vi "Volt Reader Trigger12.vi"() -> ()   [LabVIEW 2014]
uses:
  Enum State Machine Typedef.ctl
  <vilib>/Utility/error.llb/DialogType.ctl
  <vilib>/_DAQmxBase/Internals/DAQmxBase Create Channel (AI-Voltage-Basic).vi
  <vilib>/_DAQmxBase/Internals/DAQmxBase Timing (Sample Clock).vi
  <vilib>/measure/mamon.llb/Trigger Detection for 1 Channel.vi
  <vilib>/_DAQmxBase/Internals/DAQmxBase Read (Analog 2D DBL NChan NSamp).vi
  <vilib>/measure/NI_MAPro.lvlib
panel:
  out "Raw Graph":waveform(dbl)(graph)
  in  "Center":bool
  in  "Offset (percent of buffer)":dbl(knob) scale=-50.0..50.0
  out "State":T1
  out "Waveform Graph":waveform(dbl)(graph)
  in  "Buffer (Seconds)":dbl
  out "Threshold":dbl
  in  "units":i32(ring)=10348 items=["Volts"=10348, "From Custom Scale"=10065]
  in  "stop":bool
  in  "physical channels":tag
  in  "maximum value":dbl=5.0 format="%0.2f"
  in  "minimum value":dbl=-5.0 format="%0.2f"
  in  "rate":i32=1000 caption="Sample Rate"
  # "The inputs above MUST BE\nPreset before running"
  # "NOTE: Just change the Y axis value"
  # "Make Sure that Buffer does not equal 0"
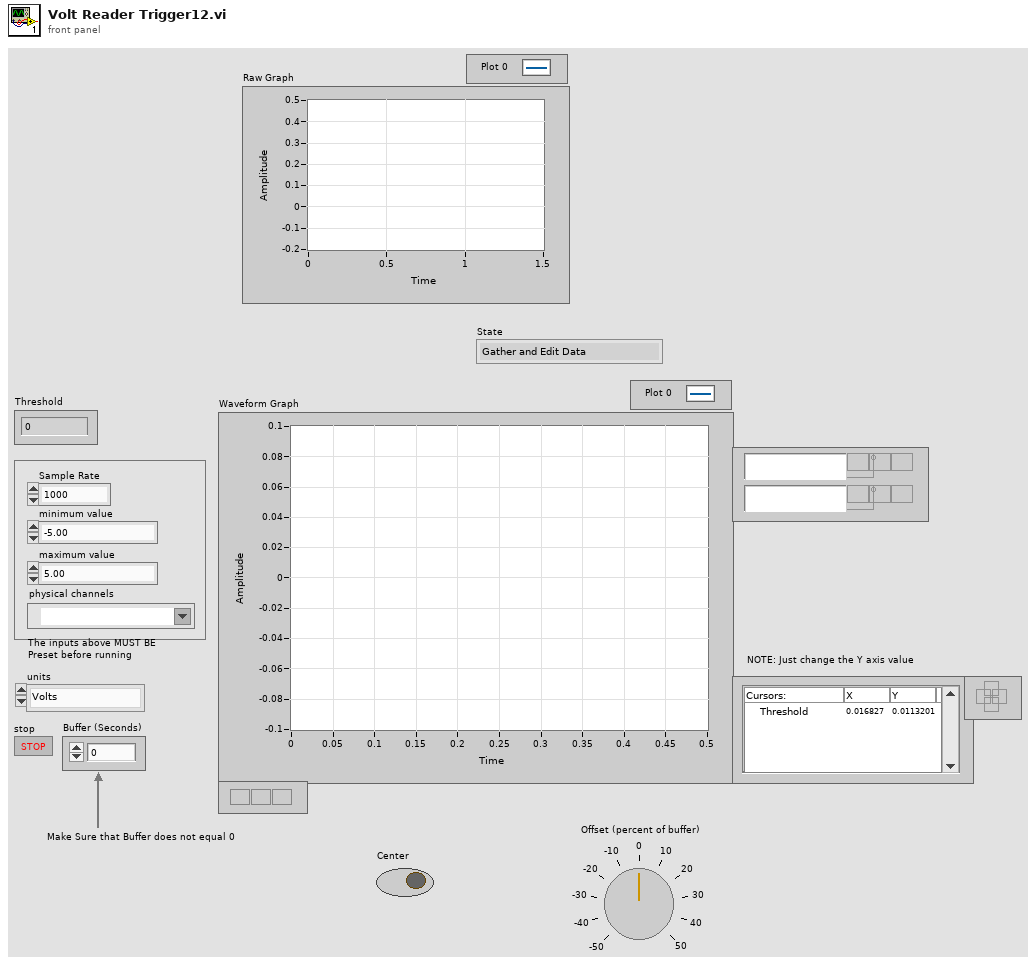
[diagram p1: front panel]
types:
  T1 = typedef "Enum State Machine Typedef.ctl" = enum16{"Gather and Edit Data", "Trigger Occured", "Just Displayed"}
  T2 = typedef "DialogType.ctl" = u16
  T3 = typedef "LVCursorListTypeDef.ctl" = cluster{"Name":string, "Color":u32, "Style":u8, "Point Style":u8, "Name Visible":bool, "Allow Drag":bool, "Cursor Mode":u32, "Plot":i32, "Index":i32, "Position":cluster{"X":dbl, "Y":dbl}, "X Scale":u32, "Y Scale":u32, "Watch Plots":i32[], "Watch All Plots":bool, "Plot Area":i32, "Label Offset":cluster{"X":dbl, "Y":dbl}}[]
  T4 = cluster{"Name":string, "Color":u32, "Style":u8, "Point Style":u8, "Name Visible":bool, "Allow Drag":bool, "Cursor Mode":u32, "Plot":i32, "Index":i32, "Position":cluster{"X":dbl, "Y":dbl}, "X Scale":u32, "Y Scale":u32, "Watch Plots":i32[], "Watch All Plots":bool, "Plot Area":i32, "Label Offset":cluster{"X":dbl, "Y":dbl}}
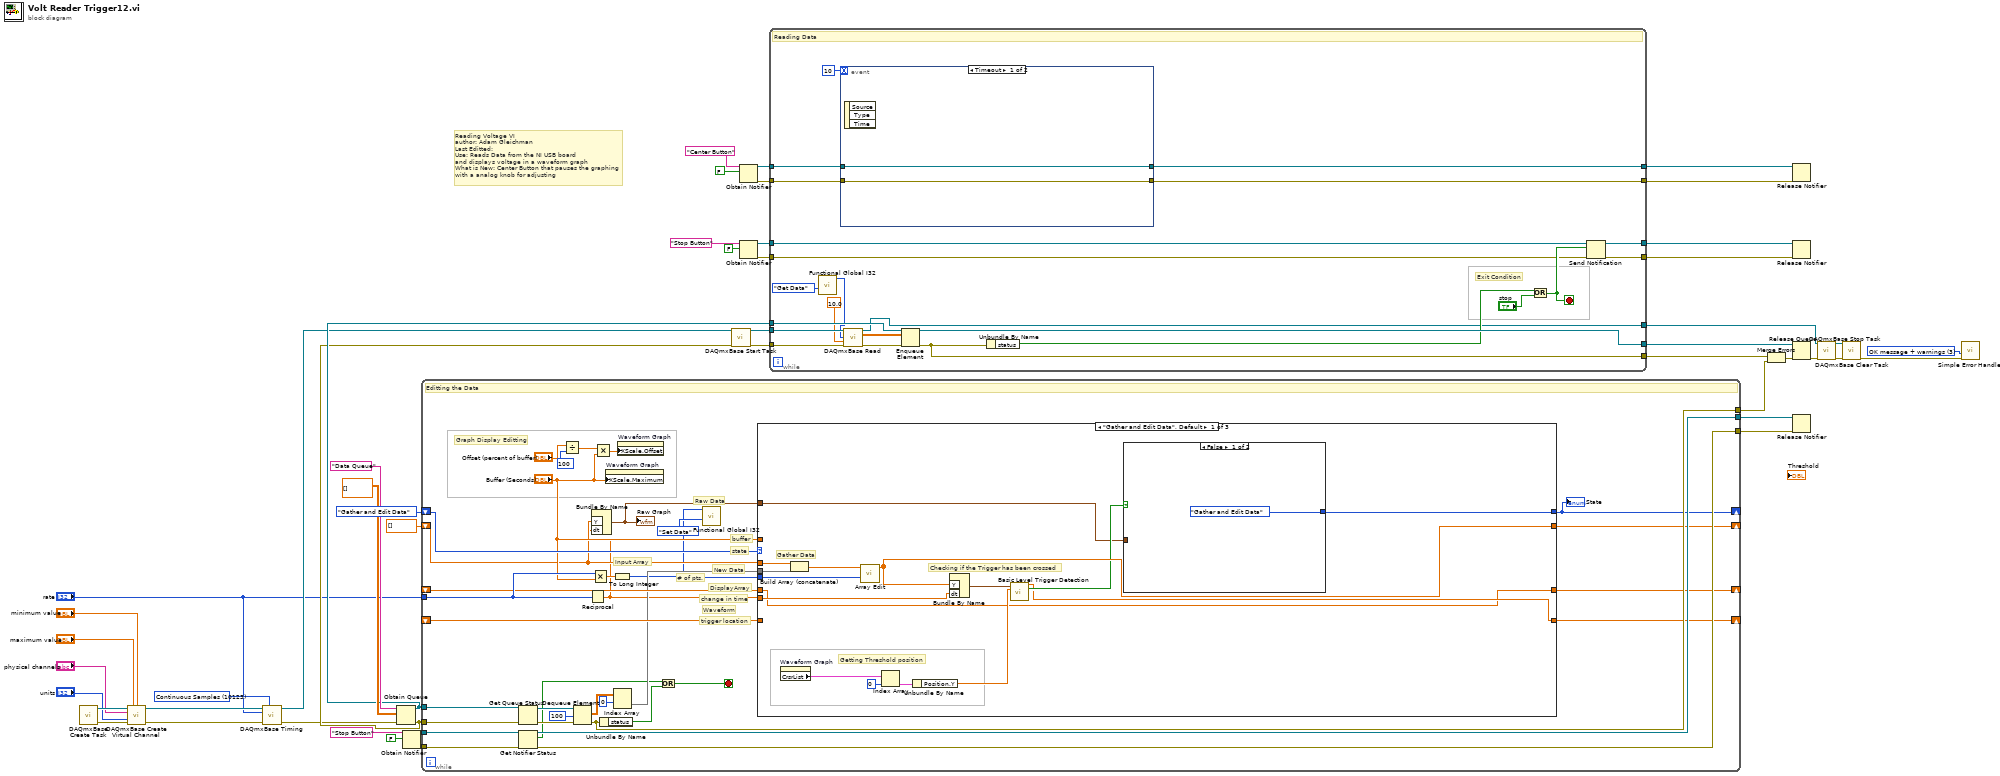
[diagram p0: block diagram]
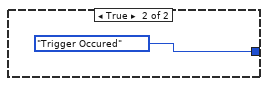
[diagram p2: hidden frame]
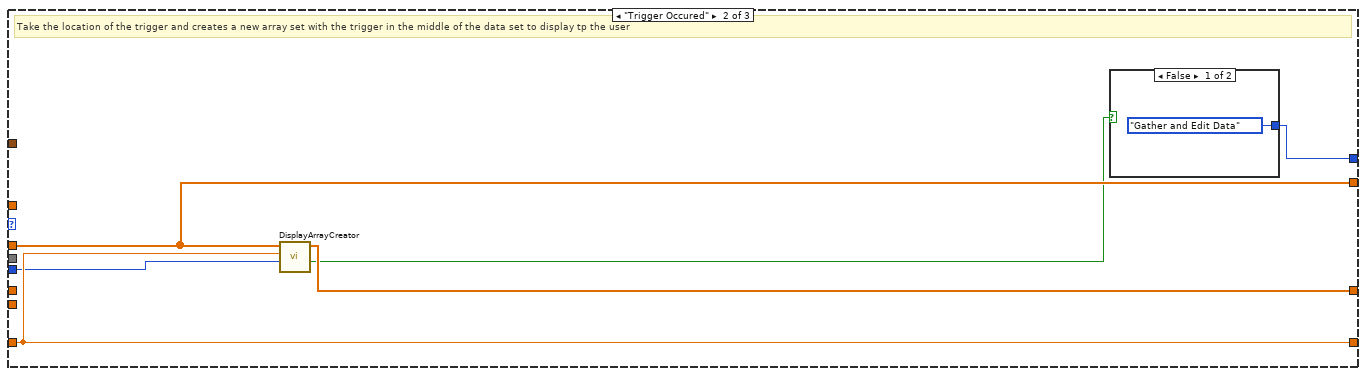
[diagram p3: hidden frame]
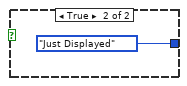
[diagram p4: hidden frame]
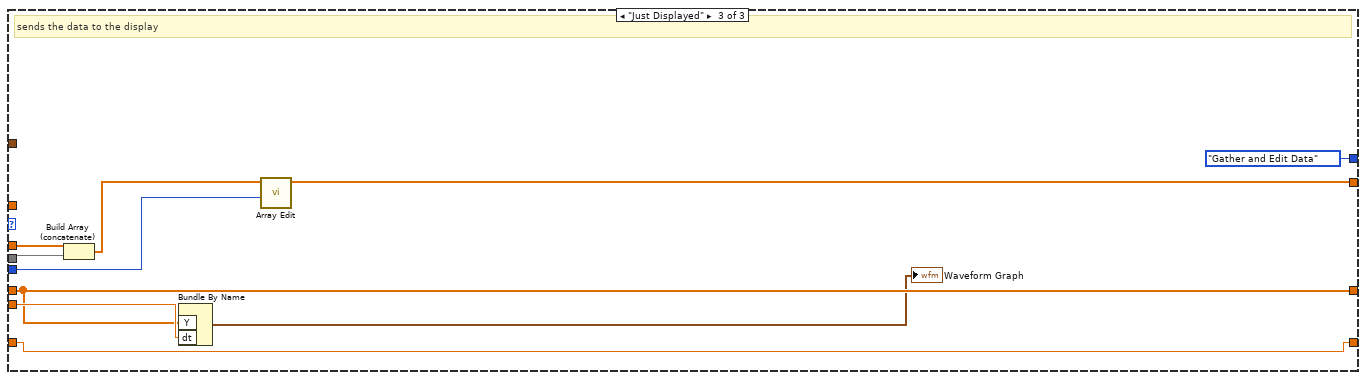
[diagram p5: hidden frame]
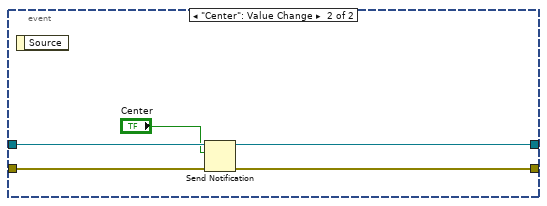
[diagram p6: hidden frame]
diagram:
  w25 = 10123 items=["Finite Samples"=10178, "Continuous Samples"=10123, "Hardware Timed Single Point"=12522] ("sample mode")
  w27 = T2 3 items=["no dialog", "OK message", "continue or stop message", "OK message + warnings", "continue/stop + warnings"] ("type of dialog (OK msg:1)")
  # "Reading Voltage VI\nauthor: Adam Gleichman\nLast Editted: \nUse: Reads Data from the NI USB board\nand displays voltage in a waveform graph\nWhat is New: Center Button that pauses the graphing\nwith a analog knob for adjusting"
  n1 = call <vilib>:"DAQmxBase Create Task.vi"() -> ("task out"=w47:refnum<k21>, "error out"=w46:errorcluster)  [unwired: 5 in, 9 out]
  n2 = call-poly <vilib>:"DAQmxBase Create Virtual Channel.vi"("task in"=w47, "maximum value"="maximum value", "minimum value"="minimum value", "physical channels"="physical channels", "units"="units", "error in"=w46) -> ("task out"=w44:refnum<k21>, "error out"=w45:errorcluster)  [unwired: 3 in, 5 out]
  n3 = call-poly <vilib>:"DAQmxBase Timing.vi"("task/channels in"=w44, "sample mode"=w25, "rate"="rate", "error in"=w45) -> ("task out"=w13:refnum<k21>, "error out"=w12:errorcluster)  [unwired: 3 in, 7 out]
  n4 = Obtain Queue(name (unnamed)="Data Queue", element data type=dbl[][] [] ("data"), error in (no error)=w12) -> (queue out=w34:refnum<queue>, error out=w33:errorcluster)  [unwired: 2 in, 1 out]
  n5 = Obtain Notifier(name (unnamed)="Stop Button", notification data type=FALSE) -> (notifier out=w18:refnum<notifier>, error out=w16:errorcluster)  [unwired: 2 in, 1 out]
  n6 = while {
    tunnel: w34 -> [w83]
    tunnel: w33 -> [w74]
    tunnel: [w81] -> w32
    tunnel: w18 -> [w79]
    tunnel: w16 -> [w78]
    tunnel: [w77] -> w14
    tunnel: [w76] -> w15
    tunnel: "rate" -> [w70]
    shift-right: [w52] -> _
    shift-left: dbl[] [] -> [w56]
    shift-right: [w51] -> _
    shift-left: Enum_State_Machine_Typedef."Gather and Edit Data" -> [w67]
    shift-right: [w50] -> _
    shift-left: _ -> [w68]
    shift-right: [w66] -> _
    shift-left: _ -> [w65]
    stop <- w80 stop-if-true
    # "Raw Data"
    # "state"
    # "Graph Display Editting"
    # "Waveform"
    # "DisplayArray"
    # "trigger location"
    # "change in time"
    # "buffer"
    # "New Data"
    # "Input Array"
    # "# of pts."
    # "Editting the Data"
    n7 = Get Queue Status(queue=w83, error in (no error)=w74) -> (queue out=w75:refnum<queue>, error out=w73:errorcluster)  [unwired: 1 in, 6 out]
    n8 = Get Notifier Status(notifier=w79, error in (no error)=w78) -> (notifier out=w77:refnum<notifier>, current notification=w57:bool, error out=w76:errorcluster)  [unwired: 2 out]
    n9 = Divide(x="Offset (percent of buffer)", y=100) -> (x/y=w60:dbl)
    n10 = Dequeue Element(queue=w75, timeout in ms (-1)=100, error in (no error)=w73) -> (element=w71:dbl[][], error out=w81:errorcluster)  [unwired: 2 out]
    n11 = Reciprocal(x=w70) -> (1/x=w55:dbl)
    n12 = Bundle By Name("Y"=w56, "dt"=w55) -> (w49:waveform(dbl))  [unwired: 1 in]
    "Raw Graph" <- w49
    n13 = Multiply(x=w70, y="Buffer (Seconds)") -> (x*y=w69:dbl)
    n14 = Multiply(x=w60, y="Buffer (Seconds)") -> (x*y=w59:dbl)
    n15 = Unbundle By Name(w81) -> ("status"=w58:bool)
    n16 = property on="Waveform Graph" class="WFGraph (strict)"("XScale.Maximum"="Buffer (Seconds)") -> ()  [unwired: 2 in, 2 out]
    n17 = To Long Integer(number=w69) -> (32bit integer=w53:i32)
    n18 = Index Array(array=w71, index (row)=0 ("index")) -> (element=w64:dbl[])  [unwired: 1 in]
    n19 = property on="Waveform Graph" class="WFGraph (strict)"("XScale.Offset"=w59) -> ()  [unwired: 2 in, 2 out]
    n20 = Or(x=w57, y=w58) -> (x .or. y?=w80:bool)
    n21 = call "Functional Global I32.vi"("Enum"=enum16{"Set Data", "Get Data"}."Set Data", "Integer In"=w53) -> ()  [unwired: 9 in, 1 out]
    n22 = case shown="\"Gather and Edit Data\", Default" w67 {
      tunnel: w56 -> [w99 w106 w116]
      tunnel: w64 -> [w98 _ w115]
      tunnel: w55 -> [w94 _ w119]
      tunnel: w53 -> [w96 w104 w113]
      tunnel: w68 -> [w85 _ w117]
      tunnel: "Buffer (Seconds)" -> [_ _ _]
      tunnel: [w91 w105 w118] -> w66
      tunnel: w65 -> [_ w105 w118]
      tunnel: [w95 w106 w112] -> w52
      tunnel: [w90 w103 Enum_State_Machine_Typedef."Gather and Edit Data"] -> w51
      tunnel: [w85 w107 w117] -> w50
      tunnel: w49 -> [w84 _ _]
      frame "Gather and Edit Data", Default {
        # "Getting Threshold position"
        # "Checking if the Trigger has been crossed"
        # "Gather Data"
        n23 = property on="Waveform Graph" class="WFGraph (strict)"() -> ("CrsrList"=w87:T3)  [unwired: 2 in, 2 out]
        n24 = Build Array (concatenate)(w99, w98) -> (w97:dbl[])
        n25 = call "Array Edit.vi"("Number of Points"=w96, "Y-values"=w97) -> ("Editted Y Values"=w95:dbl[])  [unwired: 9 in]
        n26 = Index Array(array=w87, index=0) -> (element=w89:T4)
        n27 = Unbundle By Name(w89) -> ("Position.Y"=w86:dbl)
        n28 = Bundle By Name("Y"=w95, "dt"=w94) -> (w93:waveform(dbl))  [unwired: 1 in]
        n29 = call-poly <vilib>:"Basic Level Trigger Detection.vi"("signal in"=w93, "level"=w86) -> ("trigger location"=w91:dbl, "trigger detected?"=w92:bool)  [unwired: 11 in, 1 out]
        n30 = case shown="False" w92 {
          tunnel: [Enum_State_Machine_Typedef."Gather and Edit Data" Enum_State_Machine_Typedef."Trigger Occured"] -> w90
          tunnel: w84 -> [_ _]
          frame False {
          }
          frame True {
          }
        }
      }
      frame "Trigger Occured" {
        # "Take the location of the trigger and creates a new array set with the trigger in the middle of the data set to display tp the user"
        n31 = call "DisplayArrayCreator.vi"("Number of Points"=w104, "Location of the Trigger"=w105, "Input Y Values"=w106) -> ("Valid?"=w102:bool, "Output Y Values"=w107:dbl[])  [unwired: 7 in]
        n32 = case shown="False" w102 {
          tunnel: [Enum_State_Machine_Typedef."Gather and Edit Data" Enum_State_Machine_Typedef."Just Displayed"] -> w103
          frame False {
          }
          frame True {
          }
        }
      }
      frame "Just Displayed" {
        # "sends the data to the display"
        n33 = Build Array (concatenate)(w116, w115) -> (w114:dbl[])
        n34 = Bundle By Name("Y"=w117, "dt"=w119) -> (→"Waveform Graph":waveform(dbl))  [unwired: 1 in]
        n35 = call "Array Edit.vi"("Number of Points"=w113, "Y-values"=w114) -> ("Editted Y Values"=w112:dbl[])  [unwired: 9 in]
      }
    }
    "State" <- w51
  }
  n36 = call <vilib>:"DAQmxBase Start Task.vi"("task/channels in"=w13, "error in"=w33) -> ("task out"=w42:refnum<k21>, "error out"=w43:errorcluster)  [unwired: 12 out]
  n37 = Obtain Notifier(name (unnamed)="Center Button", notification data type=FALSE) -> (notifier out=w6:refnum<notifier>, error out=w5:errorcluster)  [unwired: 2 in, 1 out]
  n38 = Obtain Notifier(name (unnamed)="Stop Button", notification data type=FALSE) -> (notifier out=w21:refnum<notifier>, error out=w20:errorcluster)  [unwired: 2 in, 1 out]
  n39 = while "Data Reading Loop" {
    tunnel: w43 -> [w141]
    tunnel: w42 -> [w142]
    tunnel: w34 -> [w139]
    tunnel: [w136] -> w37
    tunnel: [w134] -> w36
    tunnel: [w132] -> w24
    tunnel: w21 -> [w130]
    tunnel: w20 -> [w129]
    tunnel: [w128] -> w11
    tunnel: [w127] -> w10
    tunnel: w6 -> [w126]
    tunnel: w5 -> [w125]
    tunnel: [w124] -> w2
    tunnel: [w123] -> w1
    stop <- w131 stop-if-true
    # "Exit Condition"
    # "Reading Data"
    n40 = call "Functional Global I32.vi"("Enum"=enum16{"Set Data", "Get Data"}."Get Data") -> ("Integer"=w121:i32)  [unwired: 10 in]
    n41 = event shown="[0] Timeout" {
      selector: _ -> [_ _]
      dyn-events: _ -> [_ _]
      timeout: 10 -> [_ _]
      tunnel: w126 -> [w144 w149]
      tunnel: w125 -> [w143 w148]
      tunnel: [w144 w146] -> w124
      tunnel: [w143 w145] -> w123
      event Timeout {
        n42 = event-data() -> ()  [unwired: 1 in, 3 out]
      }
      event "Center": Value Change {
        n43 = event-data() -> ()  [unwired: 1 in, 1 out]
        n44 = Send Notification(notification="Center", notifier=w149, error in (no error)=w148) -> (notifier out=w146:refnum<notifier>, error out=w145:errorcluster)
      }
    }
    n45 = call-poly <vilib>:"DAQmxBase Read.vi"("task/channels in"=w142, "number of samples per channel"=w121, "timeout"=10.0, "error in"=w141) -> ("task out"=w132:refnum<k21>, "data"=w137:dbl[][], "error out"=w140:errorcluster)  [unwired: 9 in]
    n46 = Enqueue Element(queue=w139, element=w137, error in (no error)=w140) -> (queue out=w136:refnum<queue>, error out=w134:errorcluster)  [unwired: 1 in, 1 out]
    n47 = Unbundle By Name(w134) -> ("status"=w133:bool)
    n48 = Or(x=w133, y="stop") -> (x .or. y?=w131:bool)
    n49 = Send Notification(notification=w131, notifier=w130, error in (no error)=w129) -> (notifier out=w128:refnum<notifier>, error out=w127:errorcluster)
  }
  n50 = Merge Errors(w36, w32) -> (w35:errorcluster)
  n51 = Release Notifier(notifier=w2, error in (no error)=w1) -> ()  [unwired: 1 in, 3 out]
  n52 = Release Notifier(notifier=w11, error in (no error)=w10) -> ()  [unwired: 1 in, 3 out]
  n53 = Release Queue(queue=w37, error in (no error)=w35) -> (error out=w31:errorcluster)  [unwired: 1 in, 2 out]
  n54 = Release Notifier(notifier=w14, error in (no error)=w15) -> ()  [unwired: 1 in, 3 out]
  n55 = call <vilib>:"DAQmxBase Stop Task.vi"("task/channels in"=w24, "error in"=w31) -> ("task out"=w30:refnum<k21>, "error out"=w29:errorcluster)  [unwired: 12 in]
  n56 = call <vilib>:"DAQmxBase Clear Task.vi"("task in"=w30, "error in"=w29) -> ("error out"=w28:errorcluster)  [unwired: 13 in]
  n57 = call <vilib>:"Simple Error Handler.vi"("type of dialog (OK msg:1)"=w27, "error in (no error)"=w28) -> ()  [unwired: 3 in, 5 out]
